vi "Tool - Get Parent.vi"(1 "Get ref? (t)":bool=TRUE, 3 "Generations Back (1:parent)":i32=1, 5 "error in (no error)":errorcluster) -> (14 "VI Refnum":refnum<vi>, 16 "Parent Vi Name":string, 19 "error out":errorcluster)   [LabVIEW 2015, in "TLB` Template.lvlib" / "TLB`_Dependencies.lvlib"]
uses:
  TLB`_Dependencies.lvlib
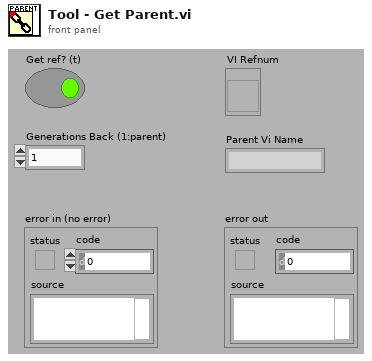
[diagram p1: front panel]
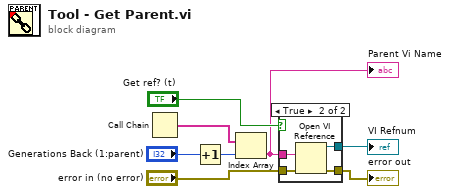
[diagram p0: block diagram]
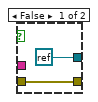
[diagram p2: hidden frame]
diagram:
  n1 = Call Chain() -> (call chain=w4:string[])
  n2 = Increment(x="Generations Back (1:parent)") -> (x+1=w1:i32)
  n3 = Index Array(array=w4, index=w1) -> (element=w6:string)
  "Parent Vi Name" <- w6
  n4 = case shown="True" "Get ref? (t)" {
    tunnel: [refnum<k0> refnum w14] -> w2
    tunnel: [w9 w13] -> w3
    tunnel: w6 -> [_ w12]
    tunnel: "error in (no error)" -> [w9 w11]
    frame False {
    }
    frame True {
      n5 = Open VI Reference(vi path=w12, error in (no error)=w11) -> (vi reference=w14:refnum<vi>, error out=w13:errorcluster)  [unwired: 4 out]
    }
  }
  "error out" <- w3
  "VI Refnum" <- w2
